vi "Publish DP Indicators.vi"   [LabVIEW 2017, in "TagDB RefManager.lvlib"]
uses:
  TagDB RefManager.lvlib
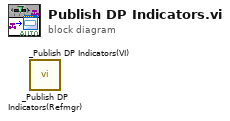
[diagram p0: block diagram]
diagram:
  n1 = call "_Publish DP Indicators(Refmgr).vi"() -> ()  [unwired: 9 in, 3 out]
  n2 = call "_Publish DP Indicators(VI).vi"() -> ()  [unwired: 9 in, 3 out]
